vi "Port.vi"(8 "error in (no error)":errorcluster, 11 "Node Ptr":T1 format="%.0x") -> (0 "error out":errorcluster)   [LabVIEW 2020, in "Communication Bus Template System Explorer.lvlib"]
uses:
  <vilib>/NI VeriStand/Custom Device API/Custom Device Item Ref.ctl
  Communication Bus Template System Explorer.lvlib
  <vilib>/NI VeriStand/Custom Device API/Custom Device API.lvlib
  <vilib>/NI VeriStand/Custom Device API/Set Item Property (String).vi
  Shared/Constants.vi
  Shared/Communication Bus Template Shared.lvlib
  <vilib>/NI VeriStand/Custom Device API/Get Item Property (U32).vi
  <vilib>/NI VeriStand/Custom Device Tools/Custom Device Utility Library/Custom Device Utility Library.lvlib
  <vilib>/NI VeriStand/Custom Device Tools/Custom Device Utility Library/NI VeriStand - Search for Item by GUID.vi
  <vilib>/NI VeriStand/Custom Device Tools/Custom Device Utility Library/Search Direction.ctl
  <vilib>/NI VeriStand/Custom Device API/Set Item Property (U32).vi
  <vilib>/NI VeriStand/Custom Device API/Get Item Property (String).vi
panel:
  in  "Baud Rate":u32
  in  "Database":string(combo)
  in  "SHDocVw.IWebBrowser":refnum<k7>(container)
  in  "Specific Header":cluster{"Section Name":string}={"Section Name"="Specific Page Settings"}
  in  "General Header":cluster{"Section Name":string}={"Section Name"="General Page Settings"}
  in  "Description":string
  in  "Name":string
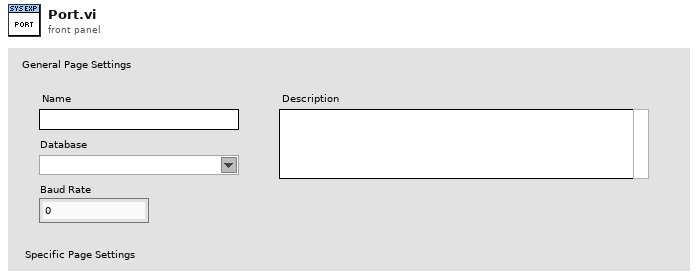
[diagram p1: front panel]
types:
  T1 = typedef "Custom Device API.lvlib/Custom Device Item Ref.ctl" = u64
  T2 = typedef "Custom Device Utility Library.lvlib/Search Direction.ctl" = enum16{"Down", "Up"}
  T3 = typedef "Custom Device API.lvlib/Custom Device Item Info.ctl" = cluster{"Name":string, "Is Channel":bool, "GUID":string, "Is Waveform":bool}
  T4 = typedef "Custom Device API.lvlib/Custom Device Commands.ctl" = enum16{"Default", "Item renamed", "Shutdown", "Dynamic button pressed"}
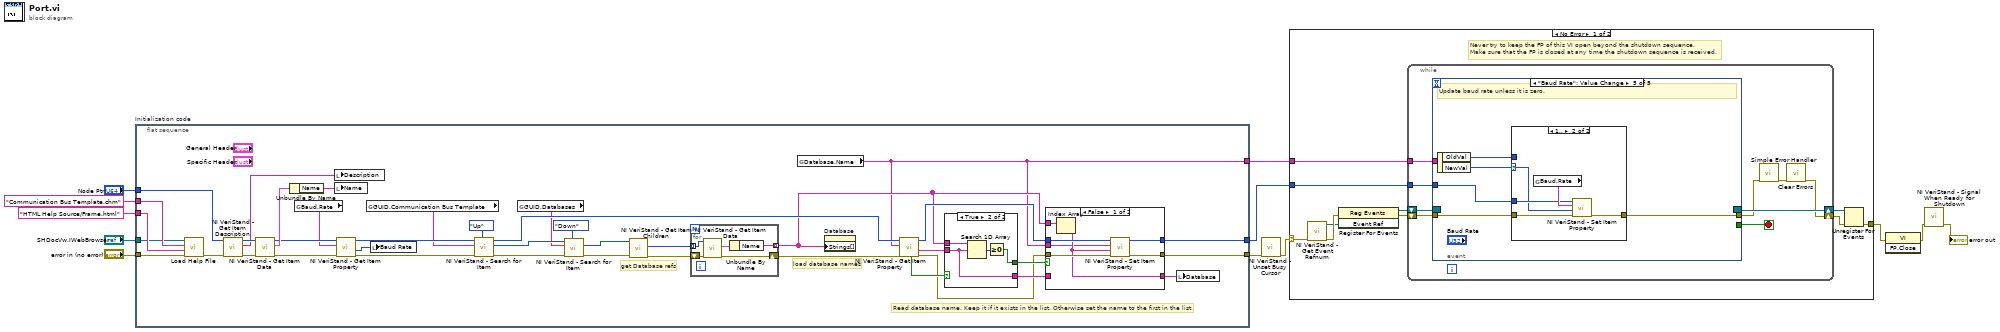
[diagram p0: block diagram]
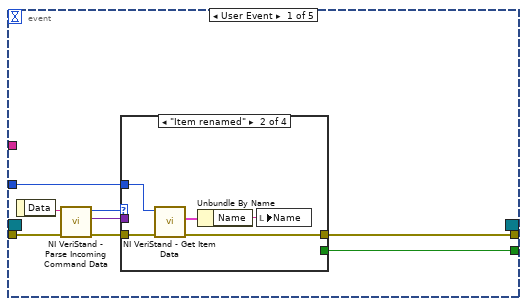
[diagram p2: hidden frame]
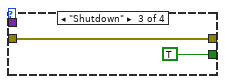
[diagram p4: hidden frame]
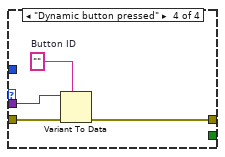
[diagram p5: hidden frame]
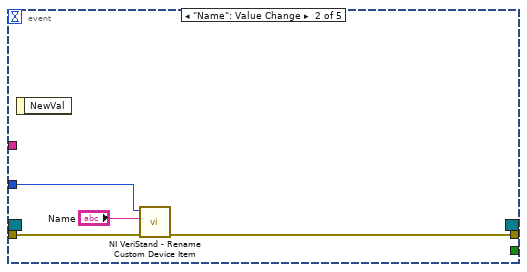
[diagram p6: hidden frame]
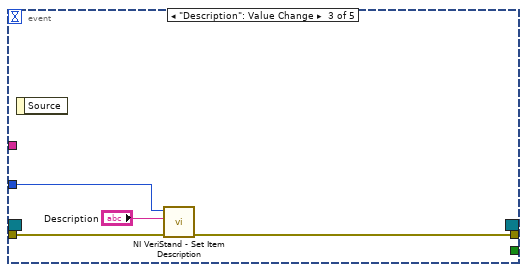
[diagram p7: hidden frame]
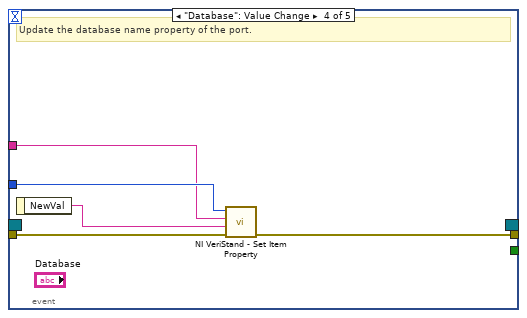
[diagram p8: hidden frame]
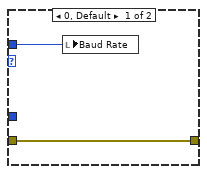
[diagram p9: hidden frame]
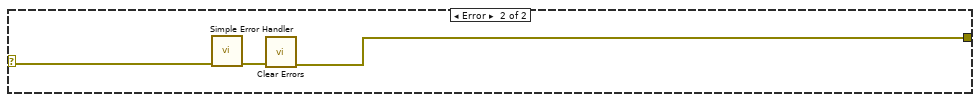
[diagram p10: hidden frame]
diagram:
  n1 = flat-sequence "Initialization code" {
    tunnel: "error in (no error)" -> [w46]
    tunnel: "Node Ptr" -> [w49]
    tunnel: [w41] -> w8
    tunnel: [w40] -> w5
    tunnel: "SHDocVw.IWebBrowser" -> [w42]
    tunnel: "HTML Help Source/Frame.html" ("CD_CHM_Section") -> [w44]
    tunnel: "Communication Bus Template.chm" ("CD_CHM_FileName") -> [w43]
    tunnel: [w14] -> w1
    frame #0 {
      # "Read database name. Keep it if it exists in the list. Otherwise set the name to the first in the list."
      # "load database names"
      # "get Database refs"
      n2 = call "Load Help File.vi"("error in (no error)"=w46, "HTML File to Load"=w44, "Main CHM File"=w43, "Browser"=w42) -> ("error out"=w45:errorcluster)  [unwired: 7 in]
      n3 = call <vilib>:"NI VeriStand - Get Item Description.vi"("error in (no error)"=w45, "Item Ref in"=w49) -> ("error out"=w51:errorcluster, "Description"=w47:string, "Item Ref out"=w52:T1)  [unwired: 7 out]
      n4 = call <vilib>:"NI VeriStand - Get Item Data.vi"("error in (no error)"=w51, "Item Ref in"=w52) -> ("error out"=w25:errorcluster, "Item Info"=w50:T3, "Item Ref out"=w23:T1)  [unwired: 7 out]
      n5 = Unbundle By Name(w50) -> ("Name"=w48:string)
      n6 = global read "Constants.vi" "Baud.Rate"() -> (w22:string)
      n7 = local write "Description"(w47) -> ()
      n8 = local write "Name"(w48) -> ()
      n9 = call-poly <vilib>:"NI VeriStand - Get Item Property.vi"("error in (no error)"=w25, "Property Name"=w22, "Item Ref in"=w23) -> ("error out"=w24:errorcluster, "Value"=w20:u32, "Item Ref out"=w21:T1)  [unwired: 5 in, 1 out]
      n10 = global read "Constants.vi" "GUID.Communication Bus Template"() -> (w19:string)
      n11 = local write "Baud Rate"(w20) -> ()
      n12 = call-poly <vilib>:"NI VeriStand - Search for Item.vi"("Direction (Down)"=Search_Direction."Up", "error in"=w24, "Item GUID"=w19, "Section Ref in"=w21) -> ("error out"=w33:errorcluster, "Item Ref"=w34:T1, "Section Ref out"=w35:T1)  [unwired: 4 in, 1 out]
      n13 = global read "Constants.vi" "GUID.Databases"() -> (w17:string)
      n14 = call-poly <vilib>:"NI VeriStand - Search for Item.vi"("Direction (Down)"=Search_Direction."Down", "error in"=w33, "Item GUID"=w17, "Section Ref in"=w34) -> ("error out"=w32:errorcluster, "Item Ref"=w31:T1)  [unwired: 4 in, 2 out]
      n15 = call <vilib>:"NI VeriStand - Get Item Children.vi"("error in (no error)"=w32, "Item Ref in"=w31) -> ("error out"=w29:errorcluster, "Child Refs"=w30:T1[])  [unwired: 6 in, 2 out]
      n16 = for {
        tunnel: w30 -> [w56] mode=indexing
        shift-right: [w54] -> w28
        shift-left: w29 -> [w55]
        tunnel: [w53] -> w16 mode=indexing
        n17 = call <vilib>:"NI VeriStand - Get Item Data.vi"("error in (no error)"=w55, "Item Ref in"=w56) -> ("error out"=w54:errorcluster, "Item Info"=w57:T3)  [unwired: 6 in, 2 out]
        n18 = Unbundle By Name(w57) -> ("Name"=w53:string)
      }
      n19 = global read "Constants.vi" "Database.Name"() -> (w14:string)
      n20 = property on="Database" class="CmbBox"("Strings[]"=w16) -> ()  [unwired: 2 in, 2 out]
      n21 = call-poly <vilib>:"NI VeriStand - Get Item Property.vi"("error in (no error)"=w28, "Property Name"=w14, "Item Ref in"=w35) -> ("error out"=w15:errorcluster, "Value"=w37:string, "Item Ref out"=w39:T1, "Found?"=w38:bool)  [unwired: 5 in]
      n22 = case shown="True" w38 {
        selector: w38 -> [w68 _]
        tunnel: w37 -> [_ w70]
        tunnel: [w68 w71] -> w36
        tunnel: [_ w70] -> w26
        tunnel: w16 -> [_ w69]
        frame False {
        }
        frame True {
          n23 = Search 1D Array(1D array=w69, element=w70) -> (index of element=w72:i32)  [unwired: 1 in]
          n24 = Greater Or Equal To 0?(x=w72) -> (x >= 0?=w71:bool)
        }
      }
      n25 = case shown="False" w36 {
        tunnel: [w64 w66] -> w41
        tunnel: [w63 w67] -> w40
        tunnel: w15 -> [w62 w66]
        tunnel: w39 -> [w61 w67]
        tunnel: [w60 w65] -> w27
        tunnel: w26 -> [_ w65]
        tunnel: w16 -> [w59 _]
        tunnel: w14 -> [w58 _]
        frame False {
          n26 = Index Array(array=w59) -> (element=w60:string)  [unwired: 1 in]
          n27 = call-poly <vilib>:"NI VeriStand - Set Item Property.vi"("error in (no error)"=w62, "Value"=w60, "Property Name"=w58, "Item Ref in"=w61) -> ("error out"=w64:errorcluster, "Item Ref out"=w63:T1)  [unwired: 5 in, 1 out]
        }
        frame True {
        }
      }
      n28 = local write "Database"(w27) -> ()
    }
  }
  n29 = call <vilib>:"NI VeriStand - Unset Busy Cursor.vi"("error in (no error)"=w8) -> ("error out"=w7:errorcluster)  [unwired: 10 out]
  n30 = case shown="No Error" w7 {
    selector: w7 -> [w74 w139]
    tunnel: [w79 w137] -> w12
    tunnel: w5 -> [w75 _]
    tunnel: w1 -> [w73 _]
    frame No Error {
      # "Never try to keep the FP of this VI open beyond the shutdown sequence.\nMake sure that the FP is closed at any time the shutdown sequence is received."
      n31 = call <vilib>:"NI VeriStand - Get Event Refnum.vi"("error in (no error)"=w74) -> ("error out"=w82:errorcluster, "Event Ref"=w78:refnum<user-event>)  [unwired: 9 out]
      n32 = register-events(error in=w82, w78) -> (reference out=w76:refnum<event-registration>, error out=w77:errorcluster)  [unwired: 1 in]
      n33 = while {
        tunnel: w75 -> [w87]
        shift-right: [w84] -> w80
        shift-left: w77 -> [w90]
        shift-right: [w91] -> w81
        shift-left: w76 -> [w89]
        tunnel: w73 -> [w83]
        stop <- w88 stop-if-true
        n34 = event shown="[4] \"Baud Rate\": Value Change" {
          selector: w89 -> [_ _ _ _ _]
          dyn-events: [_ _ _ _ _] -> w91
          timeout: _ -> [_ _ _ _ _]
          tunnel: w90 -> [w99 w115 w118 w123 w129]
          tunnel: [w95 _ _ _ _] -> w88
          tunnel: [w94 w114 w117 w122 w127] -> w86
          tunnel: w87 -> [w93 w113 w119 w124 w126]
          tunnel: w83 -> [_ _ _ w120 _]
          event User Event {
            n35 = event-data() -> ("Data"=w98:string)  [unwired: 1 out]
            n36 = call <vilib>:"NI VeriStand - Parse Incoming Command Data.vi"("error in (no error)"=w99, "Incoming data"=w98) -> ("error out"=w97:errorcluster, "Outgoing data"=w92:variant, "Action"=w96:T4)  [unwired: 7 out]
            n37 = case shown="\"Item renamed\"" w96 {
              tunnel: w97 -> [w100 w105 w106 w111]
              tunnel: [_ _ TRUE _] -> w95
              tunnel: [w100 w102 w106 w108] -> w94
              tunnel: w93 -> [_ w104 _ _]
              tunnel: w92 -> [_ _ _ w110]
              frame "Default", Default {
              }
              frame "Item renamed" {
                n38 = call <vilib>:"NI VeriStand - Get Item Data.vi"("error in (no error)"=w105, "Item Ref in"=w104) -> ("error out"=w102:errorcluster, "Item Info"=w103:T3)  [unwired: 8 out]
                n39 = Unbundle By Name(w103) -> ("Name"=w101:string)
                n40 = local write "Name"(w101) -> ()
              }
              frame "Shutdown" {
              }
              frame "Dynamic button pressed" {
                w109 = ""  # Button ID
                n41 = Variant To Data(error in=w111, type=w109, Variant=w110) -> (error out=w108:errorcluster)  [unwired: 1 out]
              }
            }
          }
          event "Name": Value Change {
            n42 = event-data() -> ()  [unwired: 2 out]
            n43 = call <vilib>:"NI VeriStand - Rename Custom Device Item.vi"("error in (no error)"=w115, "New Name"="Name", "Item Ref in"=w113) -> ("error out"=w114:errorcluster)  [unwired: 1 in, 7 out]
          }
          event "Description": Value Change {
            n44 = event-data() -> ()  [unwired: 2 out]
            n45 = call <vilib>:"NI VeriStand - Set Item Description.vi"("error in (no error)"=w118, "Description"="Description", "Item Ref in"=w119) -> ("error out"=w117:errorcluster)  [unwired: 8 out]
          }
          event "Database": Value Change {
            # "Update the database name property of the port."
            n46 = event-data() -> ("NewVal"=w121:string)  [unwired: 1 out]
            n47 = call-poly <vilib>:"NI VeriStand - Set Item Property.vi"("error in (no error)"=w123, "Value"=w121, "Property Name"=w120, "Item Ref in"=w124) -> ("error out"=w122:errorcluster)  [unwired: 5 in, 2 out]
          }
          event "Baud Rate": Value Change {
            # "Update baud rate unless it is zero."
            n48 = event-data() -> ("OldVal"=w125:u32, "NewVal"=w128:u32)  [unwired: 1 out]
            n49 = case shown="1.." w128 {
              selector: w128 -> [_ w132]
              tunnel: w129 -> [w131 w135]
              tunnel: [w131 w134] -> w127
              tunnel: w126 -> [_ w133]
              tunnel: w125 -> [w130 _]
              frame 0, Default {
                n50 = local write "Baud Rate"(w130) -> ()
              }
              frame 1.. {
                n51 = global read "Constants.vi" "Baud.Rate"() -> (w136:string)
                n52 = call-poly <vilib>:"NI VeriStand - Set Item Property.vi"("error in (no error)"=w135, "Value"=w132, "Property Name"=w136, "Item Ref in"=w133) -> ("error out"=w134:errorcluster)  [unwired: 5 in, 2 out]
              }
            }
          }
        }
        n53 = call <vilib>:"Simple Error Handler.vi"("error in (no error)"=w86) -> ("error out"=w85:errorcluster)  [unwired: 1 in, 7 out]
        n54 = call <vilib>:"Clear Errors.vi"("error in (no error)"=w85) -> ("error out"=w84:errorcluster)  [unwired: 1 in, 5 out]
      }
      n55 = Unregister For Events(event registration refnum=w81, error in=w80) -> (error out=w79:errorcluster)
    }
    frame Error {
      n56 = call <vilib>:"Simple Error Handler.vi"("error in (no error)"=w139) -> ("error out"=w138:errorcluster)  [unwired: 1 in, 7 out]
      n57 = call <vilib>:"Clear Errors.vi"("error in (no error)"=w138) -> ("error out"=w137:errorcluster)  [unwired: 1 in, 5 out]
    }
  }
  n58 = invoke class="VI" method="FP.Close"(error in=w12) -> (error out=w11:errorcluster)  [unwired: 2 in, 2 out]
  n59 = call <vilib>:"NI VeriStand - Signal When Ready for Shutdown.vi"("error in (no error)"=w11) -> ("error out"=→"error out":errorcluster)  [unwired: 10 out]
